vi "P3060_读取U64数据.vi"(8 "错误输入":errorcluster caption="错误输入（无错误）", 10 "偏移地址":u32, 11 "句柄输入":i32) -> (0 "错误输出":errorcluster, 1 "返回值":i32, 2 "U64数据":u64, 3 "句柄输出":i32)   [LabVIEW 2010]
uses:
  dll/P3060.dll
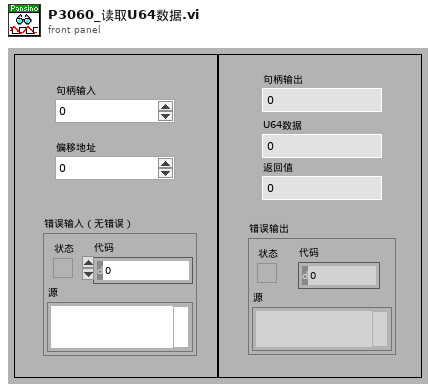
[diagram p1: front panel]
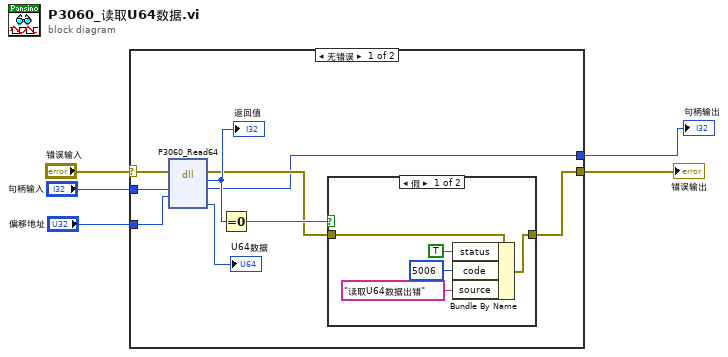
[diagram p0: block diagram]
diagram:
  n1 = case shown="无错误" "错误输入" {
    selector: "错误输入" -> [w10 w22]
    tunnel: [w14 w22] -> w3
    tunnel: "句柄输入" -> [w9 w21]
    tunnel: "偏移地址" -> [w8 _]
    tunnel: [w7 w21] -> w1
    frame No Error {
      n2 = dll-call lib="D:/driver/trunk/Drivers/P3060/P3060API/P3060APILV/Labview/P3060/_SubVI/dll/P3060.dll" fn="P3060_Read64"(error in=w10, "hDev"=w9, "Offset"=w8) -> (error out=w11:errorcluster, "return"=w13:i32, "hDev"=w7:i32, "data"=→"U64数据":u64)  [unwired: 4 in, 1 out]
      "返回值" <- w13
      n3 = Equal To 0?(x=w13) -> (x = 0?=w12:bool)
      n4 = case shown="假" w12 {
        tunnel: [w18 w20] -> w14
        tunnel: w11 -> [w19 w20]
        frame False {
          n5 = Bundle By Name(cluster=w19, "status"=TRUE, "code"=5006, "source"="读取U64数据出错") -> (w18:errorcluster)
        }
        frame True {
        }
      }
    }
    frame Error {
    }
  }
  "错误输出" <- w3
  "句柄输出" <- w1
